vi "tolerance to color converter.vi"(2 "Tolerance select":T1) -> (6 "Tolerance Color":u32(colorbox))   [LabVIEW 2018]
uses:
  tolerance--control.ctl
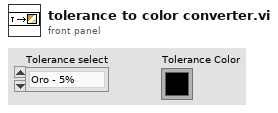
[diagram p1: front panel]
types:
  T1 = typedef "tolerance--control.ctl" = enum16{"Oro - 5%", "Plata - 10%"}
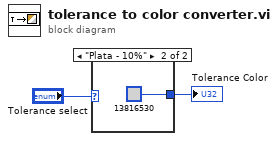
[diagram p0: block diagram]
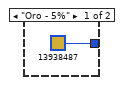
[diagram p2: hidden frame]
diagram:
  n1 = case shown="\"Plata - 10%\"" "Tolerance select" {
    tunnel: [u32 13938487 u32 13816530] -> w1
    frame "Oro - 5%" {
    }
    frame "Plata - 10%" {
    }
  }
  "Tolerance Color" <- w1
